vi "SetMeasurementMode.vi"(8 "error in (no error)":errorcluster, 9 "mode":T1(ring), 10 "Arduino Resource In":T2={"VISA resource"="", "Board Type"=enum."Uno", "Connection Type"=enum."USB / Serial", "Bytes Per Packet (15)"=15}, 11 "HMC5883L in":refnum<class "HMC5883L.lvclass">) -> (0 "error out":errorcluster, 2 "Arduino Resource Out":T2={"VISA resource"="", "Board Type"=enum."Uno", "Connection Type"=enum."USB / Serial", "Bytes Per Packet (15)"=15}, 3 "HMC5883L out":refnum<class "HMC5883L.lvclass">)   [LabVIEW 2012, in "HMC5883L.lvclass"]
uses:
  HMC5883L.lvclass
  <vilib>/LabVIEW Interface for Arduino/Type Defs/Arduino Resource.ctl
  <vilib>/LabVIEW Interface for Arduino/Type Defs/Board Type.ctl
  HMC5883L.lvclass/HMC5883L.ctl
  <vilib>/LabVIEW Interface for Arduino/LabVIEW Interface for Arduino.lvlib
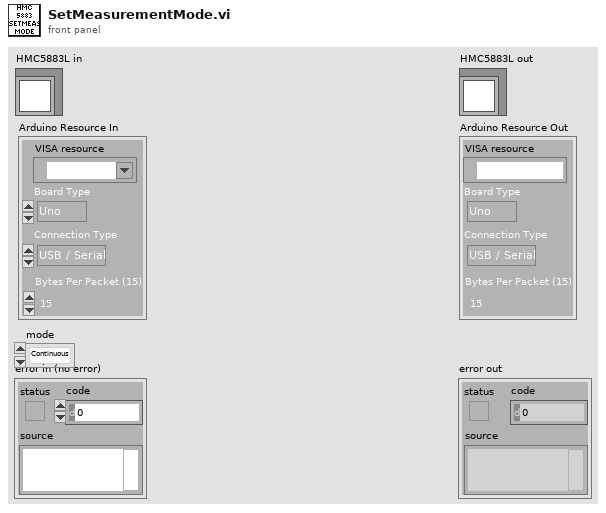
[diagram p1: front panel]
types:
  T1 = enum16{"Continuous", "SingleShot", "NoDefined", "Idle"}
  T2 = typedef "LabVIEW Interface for Arduino.lvlib/Arduino Resource.ctl" = cluster{"VISA resource":refnum<visa-resource-name>, "Board Type":T3, "Connection Type":enum8{"USB / Serial"}, "Bytes Per Packet (15)":u8}
  T3 = typedef "LabVIEW Interface for Arduino.lvlib/Board Type.ctl" = enum16{"Uno", "Dimuelanove w/Atmega 328", "Mega 2560"}
  T4 = enum16{"Continuous", "SingleShot", "NoDefined", "Idle"}[]
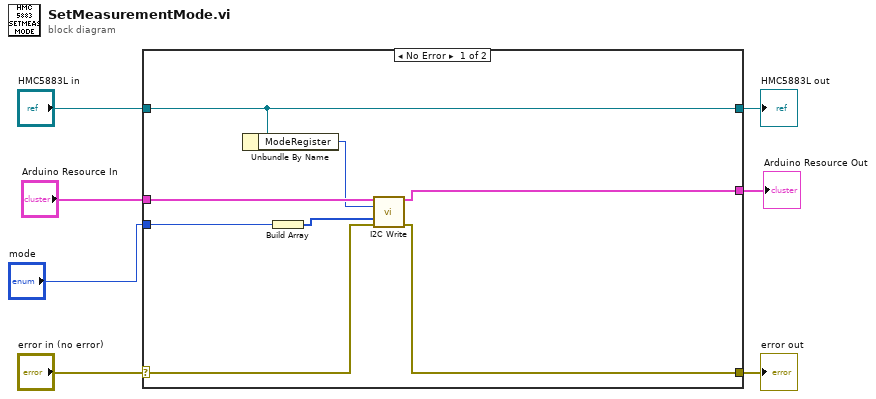
[diagram p0: block diagram]
diagram:
  n1 = case shown="No Error" "error in (no error)" {
    selector: "error in (no error)" -> [w9 w18]
    tunnel: [w8 w18] -> w6
    tunnel: [w11 w17] -> w4
    tunnel: "HMC5883L in" -> [w11 w17]
    tunnel: "mode" -> [w14 _]
    tunnel: "Arduino Resource In" -> [w13 w16]
    tunnel: [w12 w16] -> w2
    frame No Error {
      n2 = Unbundle By Name(w11) -> ("ModeRegister"=w10:u8)
      n3 = Build Array(w14) -> (w15:T4)
      n4 = call <vilib>:"I2C Write.vi"("Arduino Resource"=w13, "Address (0)"=w10, "I2C Data Bytes"=w15, "error in"=w9) -> ("Arduino Resource"=w12:T2, "error out"=w8:errorcluster)  [unwired: 10 in]
    }
    frame Error {
    }
  }
  "error out" <- w6
  "HMC5883L out" <- w4
  "Arduino Resource Out" <- w2
